vi "ASCII to U8 Array.vi"(10 "ASCII String":string) -> (2 "U8 Array":u8[](array[numeric]) format="%02x")   [LabVIEW 2025]
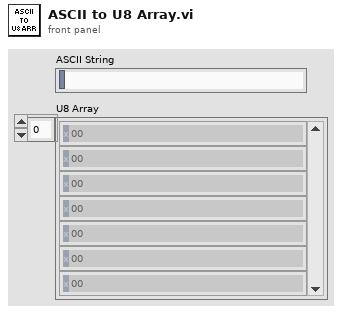
[diagram p1: front panel]
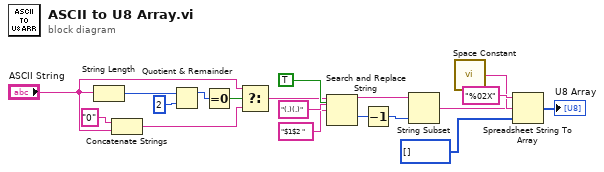
[diagram p0: block diagram]
diagram:
  n1 = String Length(string="ASCII String") -> (length=w13:i32)
  n2 = Concatenate Strings("0" ("string"), "ASCII String") -> (w8:string)
  n3 = Quotient & Remainder(x=w13, y=2) -> (x-y*floor(x/y)=w11:i32)  [unwired: 1 out]
  n4 = Equal To 0?(x=w11) -> (x = 0?=w10:bool)
  n5 = Select(t="ASCII String", s=w10, f=w8) -> (s? t:f=w7:string)
  n6 = Search and Replace String(replace all?=TRUE ("replace all? (F)"), input string=w7, search string="(.)(.)", replace string="$1$2 " ("replace string (\"\")")) -> (result string=w5:string, offset past replacement=w6:i32)  [unwired: 4 in, 2 out]
  n7 = Decrement(x=w6) -> (x-1=w3:i32)
  n8 = String Subset(string=w5, length (rest)=w3) -> (substring=w4:string)  [unwired: 1 in]
  n9 = call <vilib>:"Space Constant.vi"() -> ("String"=w14:string)
  n10 = Spreadsheet String To Array(delimiter (Tab)=w14, format string="%02X", spreadsheet string=w4, array type (2D Dbl)=u8[] []) -> (array=→"U8 Array":u8[])
